vi "Initialize Path Lookup.vi"(8 "error in (no error)":errorcluster, 11 "QControlWizard in":refnum<class "QControl Creation Wizard.lvclass">) -> (0 "error out":errorcluster, 3 "QControlWizard out":refnum<class "QControl Creation Wizard.lvclass">)   [LabVIEW 2015, in "QControl Creation Wizard.lvclass"]
uses:
  QControl Creation Wizard.lvclass
  QControl Creation Wizard.lvclass/QControl Creation Wizard.ctl
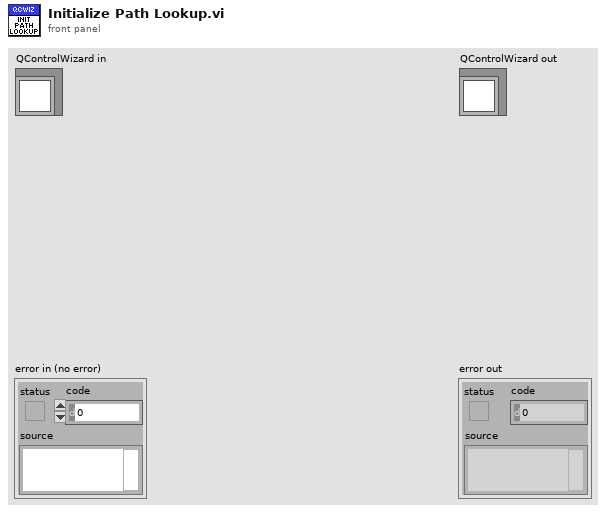
[diagram p1: front panel]
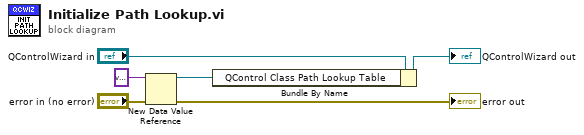
[diagram p0: block diagram]
diagram:
  n1 = New Data Value Reference(data value=variant, error in="error in (no error)") -> (data value reference=w4:refnum<data-value>, error out=→"error out":errorcluster)
  n2 = Bundle By Name(cluster="QControlWizard in", "QControl Class Path Lookup Table"=w4) -> (→"QControlWizard out":refnum<class "QControl Creation Wizard.lvclass">)
